vi "Shutdown.vi"(4 "error in (no error)":errorcluster, 7 "DeviceIOLib In":refnum<k24>) -> (0 "error out":errorcluster)   [LabVIEW 2009]
uses:
  C:/Code/Apps/Utilities/Picomotor/PicomotorApp/Install/Samples/LabVIEW/Mixed Devices/LabVIEW 2009/DeviceIOLib.dll
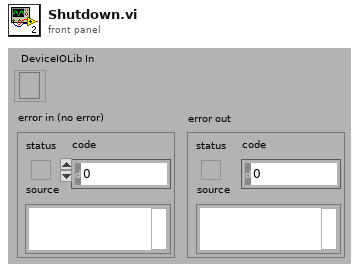
[diagram p1: front panel]
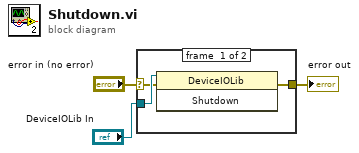
[diagram p0: block diagram]
diagram:
  n1 = case shown="No Error" "error in (no error)" {
    selector: "error in (no error)" -> [w4 w7]
    tunnel: "DeviceIOLib In" -> [w6 _]
    tunnel: [w5 w7] -> w2
    frame #0 {
      n2 = invoke class="DeviceIOLib" method="Shutdown"(reference=w6, error in=w4) -> (error out=w5:errorcluster)  [unwired: 1 in, 2 out]
    }
    frame #1 {
    }
  }
  "error out" <- w2
